vi "MockCameraToPC.vi"(8 "error in (no error)":errorcluster) -> ()   [LabVIEW 2016]
uses:
  <vilib>/Rock Robotics/WPI/Utilities/Refnum Registry Operation.ctl
  <vilib>/Rock Robotics/Network Tables/NT Write String Array.vi
  <vilib>/Rock Robotics/Network Tables/NT Write String.vi
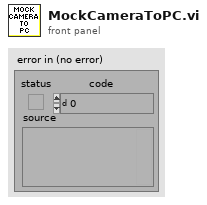
[diagram p1: front panel]
types:
  T1 = enum16{"Standard", "Buffered", "CRLF", "Immediate"}
  T2 = typedef "Refnum Registry Operation.ctl" = enum16{"set", "get", "delete", "get all names", "read name"}
  T3 = cluster{"token string":string, "token string 2":string}[]
  T4 = typedef "WPI_CameraDevRef.ctl" = cluster{"Camera Address":string, "CameraStatus":errorcluster}
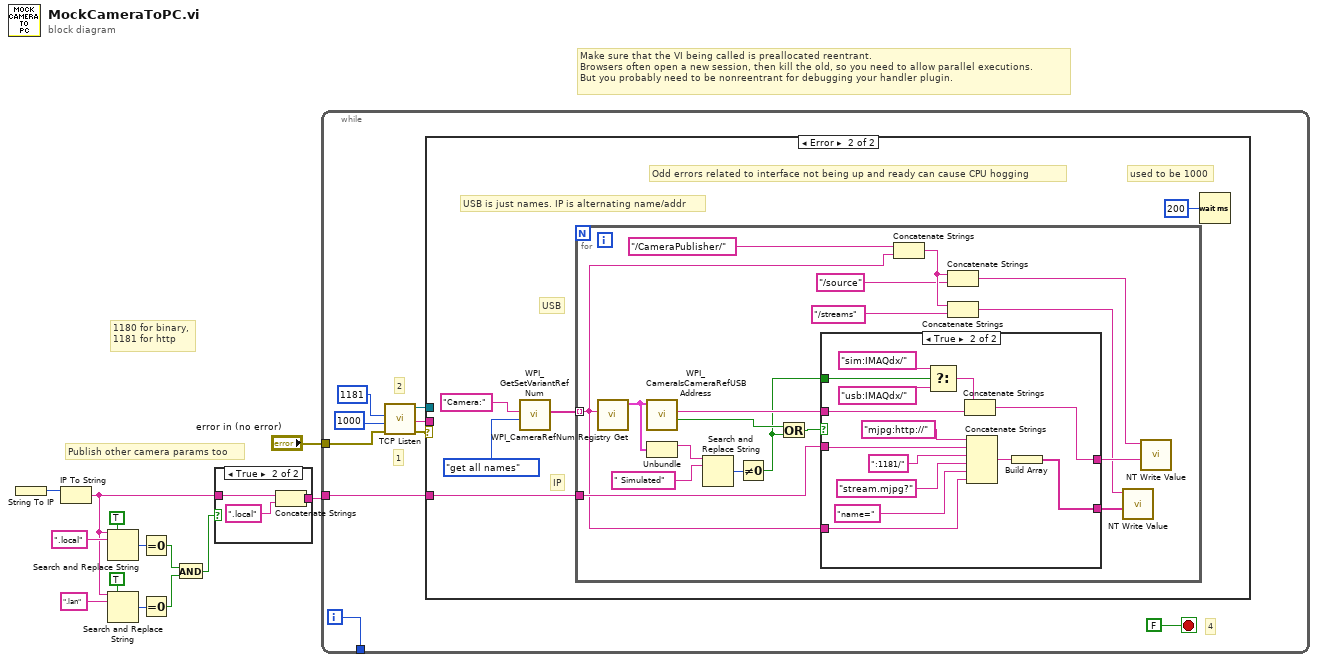
[diagram p0: block diagram]
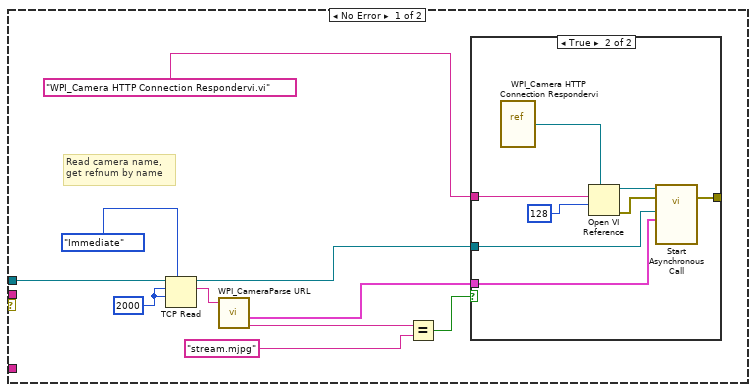
[diagram p3: hidden frame]
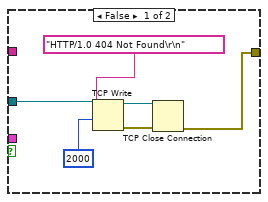
[diagram p4: hidden frame]
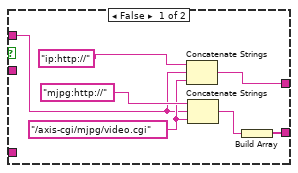
[diagram p5: hidden frame]
diagram:
  # "Make sure that the VI being called is preallocated reentrant.\nBrowsers often open a new session, then kill the old, so you need to allow parallel executions.\nBut you probably need to be nonreentrant for debugging your handler plugin."
  # "Publish other camera params too"
  # "1180 for binary,\n1181 for http"
  n1 = String To IP() -> (0:w12:u32)  [unwired: 1 in]
  n2 = IP To String(2:w12) -> (0:w1:string)  [unwired: 1 in]
  n3 = Search and Replace String(replace all?=TRUE ("replace all? (F)"), input string=w1, search string=".local") -> (number of replacements=w8:i32)  [unwired: 5 in, 3 out]
  n4 = Search and Replace String(replace all?=TRUE ("replace all? (F)"), input string=w1, search string=".lan") -> (number of replacements=w7:i32)  [unwired: 5 in, 3 out]
  n5 = Equal To 0?(x=w8) -> (x = 0?=w4:bool)
  n6 = Equal To 0?(x=w7) -> (x = 0?=w3:bool)
  n7 = And(x=w4, y=w3) -> (x .and. y?=w2:bool)
  n8 = case shown="True" w2 {
    tunnel: w1 -> [w14 w17]
    tunnel: [w14 w16] -> w11
    frame False {
    }
    frame True {
      n9 = Concatenate Strings(w17, ".local" ("string")) -> (w16:string)
    }
  }
  n10 = while {
    tunnel: "error in (no error)" -> [w25]
    tunnel: [w20] -> _
    tunnel: w11 -> [w18]
    i -> [w20]
    stop <- FALSE ("status") stop-if-true
    # "4"
    # "1"
    # "2"
    n11 = call <vilib>:"TCP Listen.vi"("error in (no error)"=w25, "timeout ms (wait forever: -1)"=u16 1000 ("port"), "port"=u16 1181) -> ("error out"=w22:errorcluster, "remote address"=w26:string, "connection ID"=w24:refnum<k5>)  [unwired: 1 in, 5 out]
    n12 = case shown="Error" w22 {
      tunnel: w26 -> [_ _]
      tunnel: w24 -> [w33 _]
      tunnel: w18 -> [_ w51]
      frame No Error {
        w34 = 2000
        # "Read camera name,\nget refnum by name"
        n13 = TCP Read(connection ID=w33, bytes to read=w34, 7:T1."Immediate" ("mode (standard)"), 9:w34) -> (connection ID out=w32:refnum<k5>, data out=w27:string)  [unwired: 1 in, 1 out]
        n14 = call <vilib>:"WPI_CameraParse URL.vi"("URL"=w27) -> ("cgi string"=w29:string, "parameters"=w28:T3)  [unwired: 7 in, 2 out]
        n15 = Equal?(x=w29, y="stream.mjpg") -> (x = y?=w31:bool)
        n16 = case shown="True" w31 {
          tunnel: "WPI_Camera HTTP Connection Respondervi.vi" -> [_ w50]
          tunnel: w32 -> [w42 w46]
          tunnel: [w37 w44] -> _
          tunnel: w28 -> [_ w43]
          frame False {
            n17 = TCP Write(connection ID=w42, data in="HTTP/1.0 404 Not Found\r\n" ("regular expression"), 9:2000) -> (connection ID out=w41:refnum<k5>, error out=w38:errorcluster)  [unwired: 1 in, 1 out]
            n18 = TCP Close Connection(connection ID=w41, error in (no error)=w38) -> (error out=w37:errorcluster)  [unwired: 2 out]
          }
          frame True {
            n19 = vi-ref <vilib>:"WPI_Camera HTTP Connection Respondervi.vi"() -> (w48:refnum<vi>)
            n20 = Open VI Reference(type specifier VI Refnum (for type only)=w48, vi path=w50, options=128) -> (vi reference=w47:refnum<vi>, error out=w45:errorcluster)  [unwired: 3 in]
            n21 = call-by-ref "Start Asynchronous Call"(reference=w47, error in=w45, "parameters"=w43, "connection ID"=w46) -> (error out=w44:errorcluster)  [unwired: 10 in, 1 out]
          }
        }
      }
      frame Error {
        # "used to be 1000"
        # "USB is just names. IP is alternating name/addr"
        # "IP"
        # "USB"
        # "Odd errors related to interface not being up and ready can cause CPU hogging"
        n22 = call <vilib>:"WPI_GetSetVariantRefNum.vi"("Operation"=Refnum_Registry_Operation."get all names" ("menu"), "refnum name"="Camera:") -> ("names"=w52:string[])  [unwired: 7 in, 2 out]
        n23 = for {
          tunnel: w52 -> [w70] mode=indexing
          tunnel: w51 -> [w73]
          n24 = call <vilib>:"WPI_CameraRefNum Registry Get.vi"("refnum name"=w70) -> ("CameraDevRef"=w61:T4)  [unwired: 9 in, 1 out]
          n25 = call <vilib>:"WPI_CameraIsCameraRefUSBAddress.vi"("CameraDevRef"=w61) -> ("USB?"=w58:bool, "Camera Address Out"=w63:string)  [unwired: 7 in, 2 out]
          n26 = Unbundle(w61) -> ("Camera Address"=w60:string)  [unwired: 1 out]
          n27 = Search and Replace String(input string=w60, search string=" Simulated") -> (number of replacements=w59:i32)  [unwired: 6 in, 3 out]
          n28 = Not Equal To 0?(x=w59) -> (x != 0?=w56:bool)
          n29 = Or(x=w58, y=w56) -> (x .or. y?=w57:bool)
          n30 = case shown="True" w57 {
            tunnel: w63 -> [w76 w86]
            tunnel: w73 -> [_ w93]
            tunnel: w70 -> [_ w89]
            tunnel: [w74 w85] -> w72
            tunnel: [w78 w87] -> w64
            tunnel: w56 -> [_ w84]
            frame False {
              w77 = "/axis-cgi/mjpg/video.cgi"
              n31 = Concatenate Strings("ip:http://", w76, w77) -> (w74:string)
              n32 = Concatenate Strings("mjpg:http://", w76, w77) -> (w79:string)
              n33 = Build Array(w79) -> (w78:string[])
            }
            frame True {
              n34 = Select(t="sim:IMAQdx/", s=w84, f="usb:IMAQdx/") -> (s? t:f=w81:string)
              n35 = Concatenate Strings(w81, w86) -> (w85:string)
              n36 = Concatenate Strings("mjpg:http://", w93, ":1181/", "stream.mjpg?", "name=", w89) -> (w88:string)
              n37 = Build Array(w88) -> (w87:string[])
            }
          }
          n38 = Concatenate Strings("/CameraPublisher/", w70) -> (w68:string)
          n39 = Concatenate Strings(w68, "/source") -> (w65:string)
          n40 = Concatenate Strings(w68, "/streams") -> (w66:string)
          n41 = call-poly <vilib>:"NT Write Value.vi"("String Array"=w64, "Name"=w66) -> ()  [unwired: 9 in, 1 out]
          n42 = call-poly <vilib>:"NT Write Value.vi"("String"=w72, "Name"=w65) -> ()  [unwired: 9 in, 1 out]
        }
        n43 = Wait (ms)(milliseconds to wait=u32 200) -> ()  [unwired: 1 out]
      }
    }
  }
